vi "Perform Action.vi"(8 "error in (no error)":errorcluster, 10 "Input":variant, 11 "object in":refnum<class "Fetch Waveforms CFG.lvclass">) -> (0 "error out":errorcluster, 2 "Output":variant, 3 "object out":refnum<class "Fetch Waveforms CFG.lvclass">)   [LabVIEW 2023, in "Scope Simulated CFGs.lvlib" / "Fetch Waveforms CFG.lvclass"]
uses:
  Fetch Waveforms CFG.lvclass
  Fetch Waveforms CFG.lvclass/Fetch Waveforms CFG.ctl
  <vilib>/measure/NI_MABase.lvlib
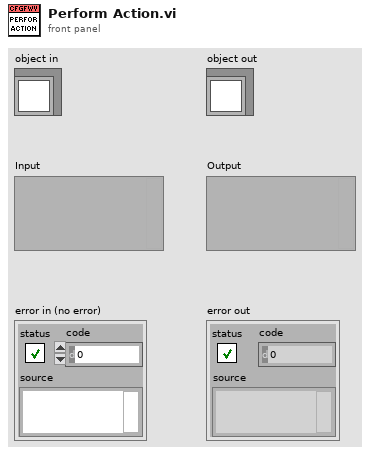
[diagram p1: front panel]
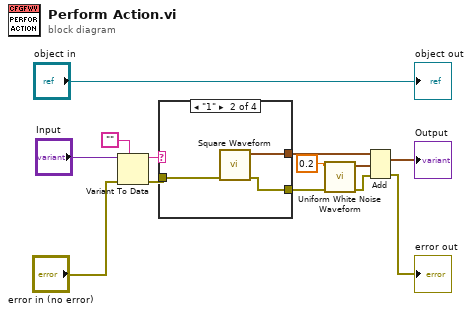
[diagram p0: block diagram]
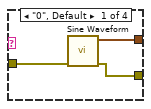
[diagram p2: hidden frame]
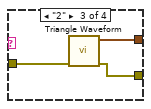
[diagram p3: hidden frame]
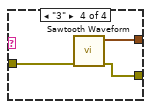
[diagram p4: hidden frame]
diagram:
  n1 = Variant To Data(error in="error in (no error)", type="", Variant="Input") -> (data=w2:string, error out=w3:errorcluster)
  n2 = case shown="\"1\"" w2 {
    tunnel: [w16 w18 w21 w25] -> w12
    tunnel: w3 -> [w15 w19 w22 w24]
    tunnel: [w14 w17 w20 w23] -> w9
    frame "0", Default {
      n3 = call <vilib>:"Sine Waveform.vi"("error in (no error)"=w15) -> ("error out"=w14:errorcluster, "signal out"=w16:waveform(dbl))  [unwired: 9 in]
    }
    frame "1" {
      n4 = call <vilib>:"Square Waveform.vi"("error in (no error)"=w19) -> ("error out"=w17:errorcluster, "signal out"=w18:waveform(dbl))  [unwired: 9 in]
    }
    frame "2" {
      n5 = call <vilib>:"Triangle Waveform.vi"("error in (no error)"=w22) -> ("error out"=w20:errorcluster, "signal out"=w21:waveform(dbl))  [unwired: 9 in]
    }
    frame "3" {
      n6 = call <vilib>:"Sawtooth Waveform.vi"("error in (no error)"=w24) -> ("error out"=w23:errorcluster, "signal out"=w25:waveform(dbl))  [unwired: 9 in]
    }
  }
  n7 = call <vilib>:"Uniform White Noise Waveform.vi"("error in (no error)"=w9, "amplitude"=0.2) -> ("error out"=w8:errorcluster, "signal out"=w11:waveform(dbl))  [unwired: 8 in]
  n8 = Add(1:w11, 2:w12, 4:w8) -> (0:→"Output":waveform(dbl), 3:→"error out":errorcluster)
  "object out" <- "object in"
